vi "ResetMissionArrays.vi"(10 "Mission Array Replacement":refnum<class "GenericMission.lvclass">[](array[class]), 11 "Mission Arrays":T1 {"Readable Missions"."Points of Interest"."North" format="%#_10f"; "Readable Missions"."Points of Interest"."East" format="%#_8f"}) -> (3 "Mission Arrays":T1 {"Readable Missions"."Points of Interest"."North" format="%#_10f"; "Readable Missions"."Points of Interest"."East" format="%#_8f"})   [LabVIEW 2013]
doc: "This VI takes in a given mission array and resets the OCU array cluster using that mission array. This is used for taking the missions from Main and resetting the OCU missions with them. It is useful when Main has been running for a while and already has missions, and you need to restart the OCU.\n\nEric Schneider, August 2014"
uses:
  TypeDef/mission_arrays.ctl
  cRIO_Code/Data/TypeDefs/MissionDescription.ctl
  cRIO_Code/Data/TypeDefs/MissionTypeControl.ctl
  cRIO_Code/Data/TypeDefs/UTM Location.ctl
  cRIO_Code/Logic/Classes/Missions/GenericMission/GenericMission.lvclass
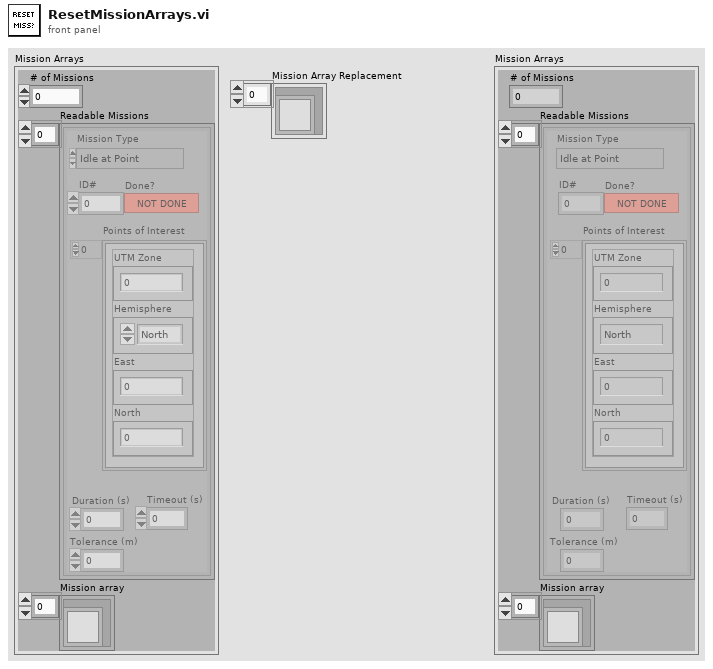
[diagram p1: front panel]
types:
  T1 = typedef "mission_arrays.ctl" = cluster{"# of Missions":i32, "Readable Missions":T2[], "Mission array":refnum<class "GenericMission.lvclass">[]}
  T2 = typedef "MissionDescription.ctl" = cluster{"Duration (s)":dbl, "Timeout (s)":dbl, "Tolerance (m)":dbl, "Mission Type":T3, "Points of Interest":T4[], "ID#":i32, "Done?":bool}
  T3 = typedef "MissionTypeControl.ctl" = enum16{"Idle at Point", "Drive to Waypoint", "Round Buoy to Port", "Round Buoy to Starboard", "Pass Between Buoys", "Station Keeping"}
  T4 = typedef "UTM Location.ctl" = cluster{"UTM Zone":dbl, "Hemisphere":enum16{"North", "South"}, "East":dbl, "North":dbl}
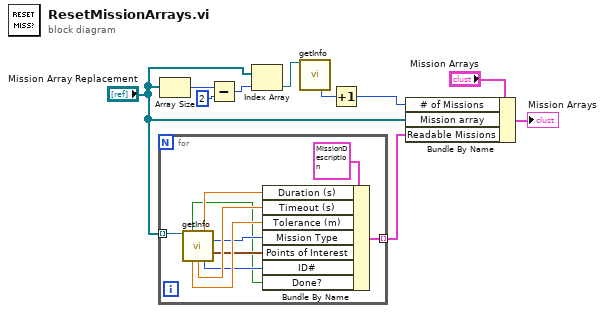
[diagram p0: block diagram]
diagram:
  n1 = for {
    tunnel: "Mission Array Replacement" -> [w19] mode=indexing
    tunnel: [w11] -> w4 mode=indexing
    n2 = call-dynamic "getInfo.vi"("GenericMission in"=w19) -> ("Done"=w12:bool, "Duration (s)"=w18:dbl, "Mission Type"=w15:T3, "Points of Interest"=w14:T4[], "Tolerance (m)"=w17:dbl, "Timeout (s)"=w16:dbl, "ID#"=w13:i16)  [unwired: 6 in, 2 out]
    n3 = Bundle By Name(cluster=T2 {"Duration (s)"=-1.0, "Timeout (s)"=-1.0, "Tolerance (m)"=0.0, "Mission Type"=enum."Idle at Point", "Points of Interest"=[], "ID#"=0, "Done?"=FALSE} ("element"), "Duration (s)"=w18, "Timeout (s)"=w16, "Tolerance (m)"=w17, "Mission Type"=w15, "Points of Interest"=w14, "ID#"=w13, "Done?"=w12) -> (w11:T2)
  }
  n4 = Array Size(array="Mission Array Replacement") -> (size(s)=w3:i32)
  n5 = Subtract(x=w3, y=2) -> (x-y=w1:i32)
  n6 = Index Array(array="Mission Array Replacement", index=w1) -> (element=w8:refnum<class "GenericMission.lvclass">)
  n7 = call-dynamic "getInfo.vi"("GenericMission in"=w8) -> ("ID#"=w7:i16)  [unwired: 6 in, 8 out]
  n8 = Increment(x=w7) -> (x+1=w6:i16)
  n9 = Bundle By Name(cluster="Mission Arrays", "# of Missions"=w6, "Mission array"="Mission Array Replacement", "Readable Missions"=w4) -> (→"Mission Arrays":T1)
